vi "setValueDH.vi"(7 "Focus":i32, 8 "error in (no error)":errorcluster, 9 "Value":string, 10 "ItemName":string, 11 "DataHandler in":refnum<class "DataHandlerMYiTOPS.lvclass">) -> (0 "error out":errorcluster, 3 "DataHandler out":refnum<class "DataHandlerMYiTOPS.lvclass">)   [LabVIEW 2015, in "DataHandlerMYiTOPS.lvclass"]
uses:
  DataHandlerMYiTOPS.lvclass
  <vilib>/drjdpowell/SQLite Library/Transaction Helpers/Transaction.lvlib
  <vilib>/drjdpowell/SQLite Library/SQLite.lvlib
  <vilib>/drjdpowell/SQLite Library/SQL Connection/Execute SQL (No results).vi
  <vilib>/drjdpowell/SQLite Library/SQL Connection/Connection.lvclass
panel:
  out "concatenated string":string
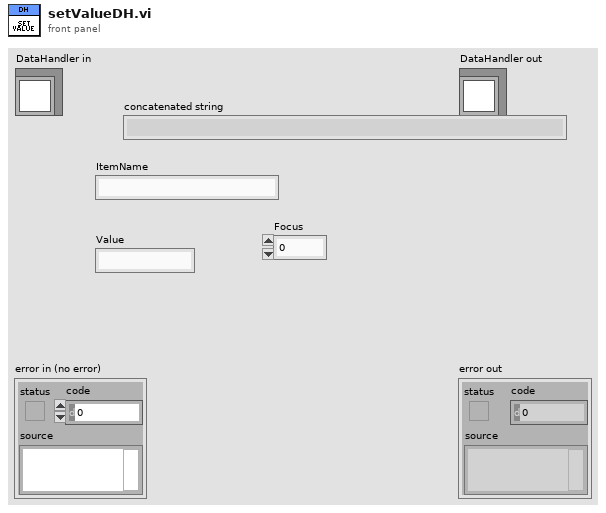
[diagram p1: front panel]
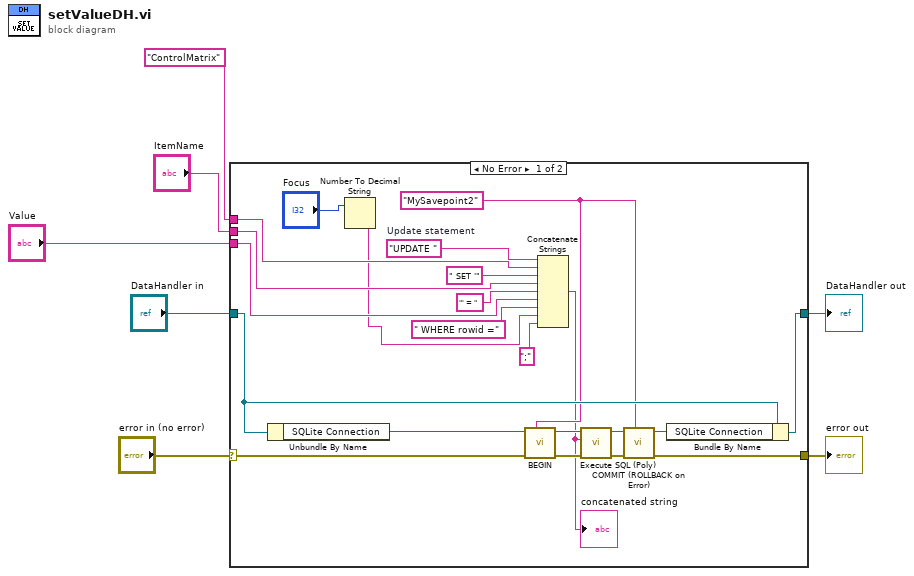
[diagram p0: block diagram]
diagram:
  n1 = case shown="No Error" "error in (no error)" {
    selector: "error in (no error)" -> [w24 w31]
    tunnel: [w23 w31] -> w6
    tunnel: [w28 w30] -> w4
    tunnel: "DataHandler in" -> [w29 w30]
    tunnel: "Value" -> [w12 _]
    tunnel: "ItemName" -> [w19 _]
    tunnel: "ControlMatrix" ("TableName") -> [w20 _]
    frame No Error {
      w17 = "MySavepoint2" ("Savepoint name")
      w22 = "UPDATE "  # Update statement
      n2 = Unbundle By Name(w29) -> ("SQLite Connection"=w27:refnum<class "Connection.lvclass">)
      n3 = Number To Decimal String(number="Focus") -> (decimal integer string=w9:string)  [unwired: 1 in]
      n4 = call <vilib>:"BEGIN.vi"("Savepoint name"=w17, "error in (no error)"=w24, "Connection in"=w27) -> ("error out"=w14:errorcluster, "Connection out"=w18:refnum<class "Connection.lvclass">)  [unwired: 7 in]
      n5 = Concatenate Strings(w22, w20, " SET '" ("string"), w19, "' = " ("string"), w12, " WHERE rowid =" ("string"), w9, ";" ("string")) -> (w13:string)
      "concatenated string" <- w13
      n6 = call-poly <vilib>:"Execute SQL (Poly).vi"("error in (no error)"=w14, "SQL"=w13, "SQLite Connection in"=w18) -> ("error out"=w15:errorcluster, "SQLite Connection out"=w16:refnum<class "Connection.lvclass">)  [unwired: 7 in]
      n7 = call <vilib>:"COMMIT (ROLLBACK on Error).vi"("Savepoint name"=w17, "error in (no error)"=w15, "Connection in"=w16) -> ("error out"=w23:errorcluster, "Connection out"=w26:refnum<class "Connection.lvclass">)  [unwired: 7 in]
      n8 = Bundle By Name(cluster=w29, "SQLite Connection"=w26) -> (w28:refnum<class "DataHandlerMYiTOPS.lvclass">)
    }
    frame Error {
    }
  }
  "error out" <- w6
  "DataHandler out" <- w4
